vi "지진계측기(교수님 코드)_AI 및 DI 추가 스위치 제어.vi"() -> ()   [LabVIEW 2021]
uses:
  <vilib>/DAQmx/read.llb/DAQmx Read (Digital U8 1Chan 1Samp).vi
  <vilib>/DAQmx/read.llb/DAQmx Read (Analog 1D DBL 1Chan NSamp).vi
  <vilib>/Analysis/baseanly.llb/Mean (DBL).vi
  <vilib>/DAQmx/create/channels.llb/DAQmx Create Channel (AI-Voltage-Basic).vi
  <vilib>/DAQmx/configure/timing.llb/DAQmx Timing (Sample Clock).vi
  <vilib>/DAQmx/create/channels.llb/DAQmx Create Channel (DI-Digital Input).vi
  <vilib>/DAQmx/miscellaneous.llb/DAQmx Fill In Error Info.vi
  <vilib>/Analysis/NI_AALBase.lvlib
panel:
  out "문자열":string
  out "알람발생":bool
  in  "시작":bool
  out "웨이브폼 차트":dbl(graph)
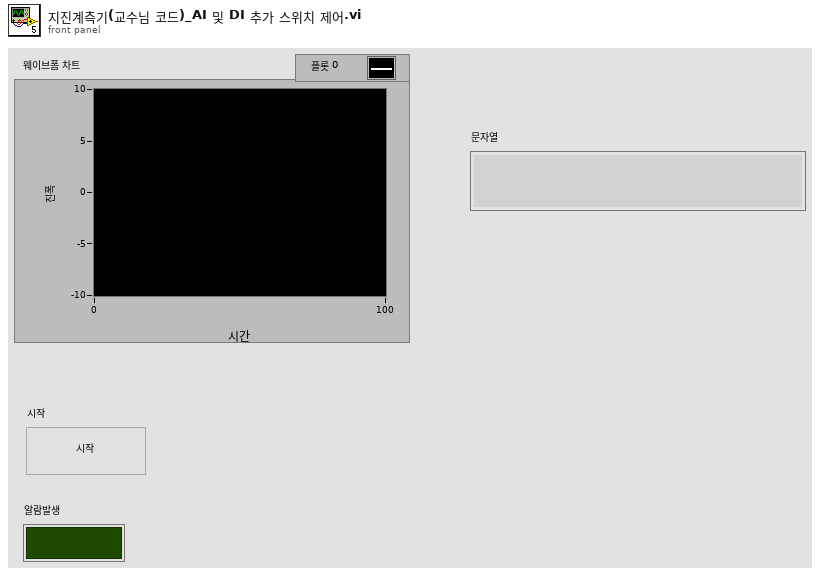
[diagram p1: front panel]
types:
  T1 = enum16{"초기화", "대기", "감지 시작", "알람 발생", "알람 리셋", "정지"}
  T2 = cluster{"AI":refnum<k21>, "DI":refnum<k21>, "알람 발생":bool, "데이터":dbl, "알람 데이터":string}
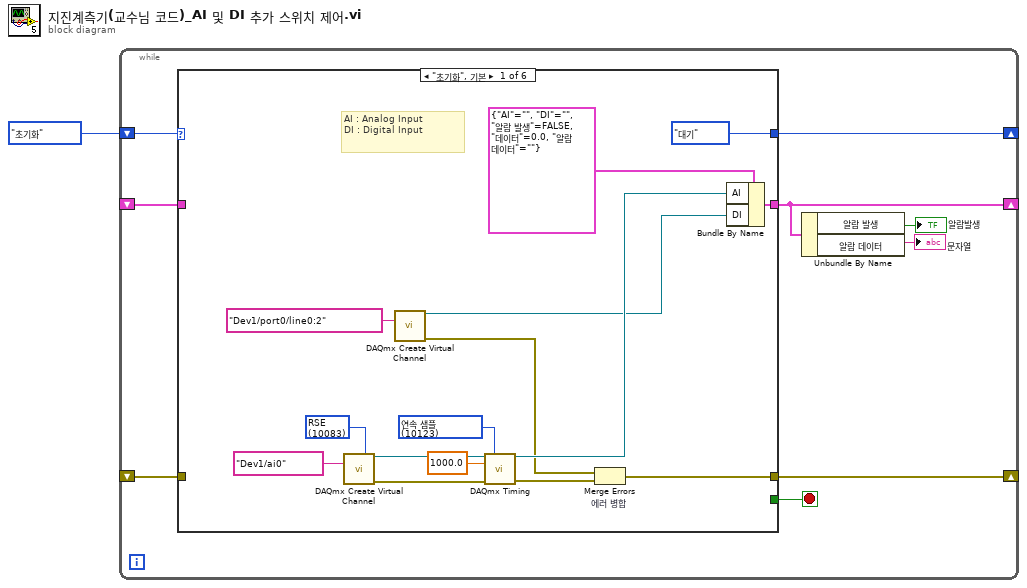
[diagram p0: block diagram]
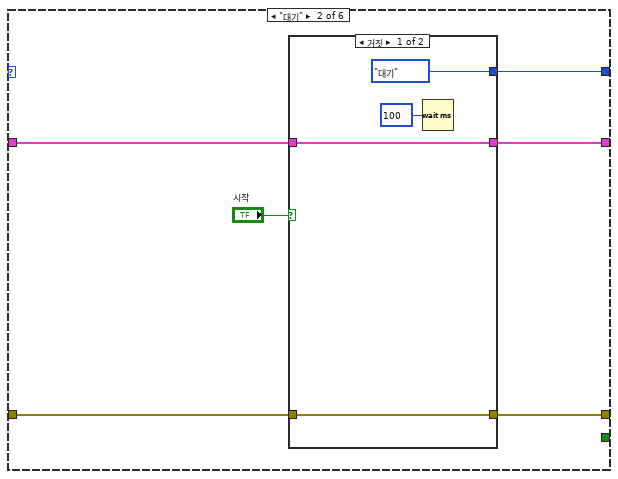
[diagram p2: hidden frame]
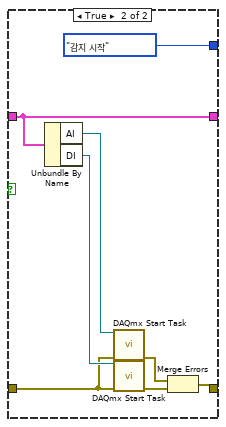
[diagram p3: hidden frame]
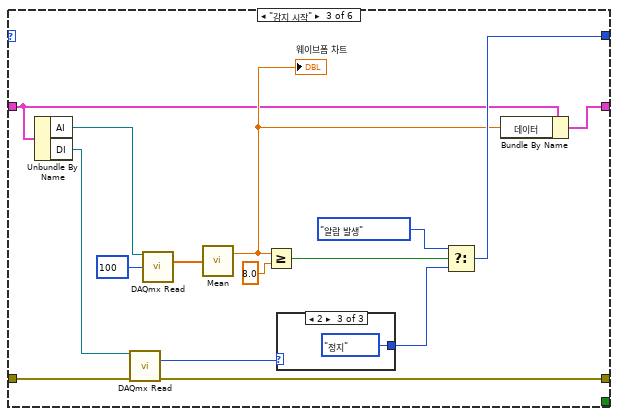
[diagram p4: hidden frame]
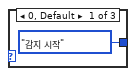
[diagram p5: hidden frame]
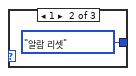
[diagram p6: hidden frame]
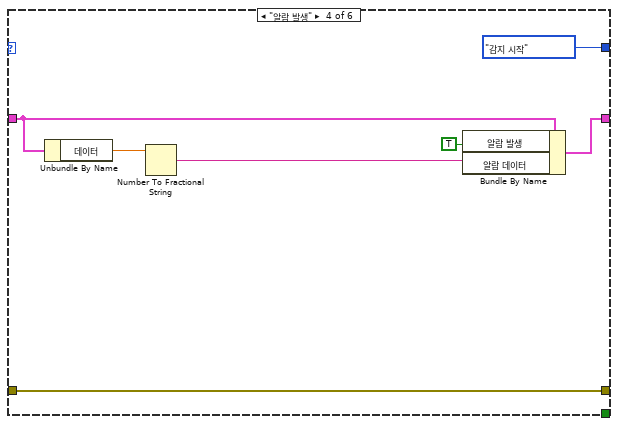
[diagram p7: hidden frame]
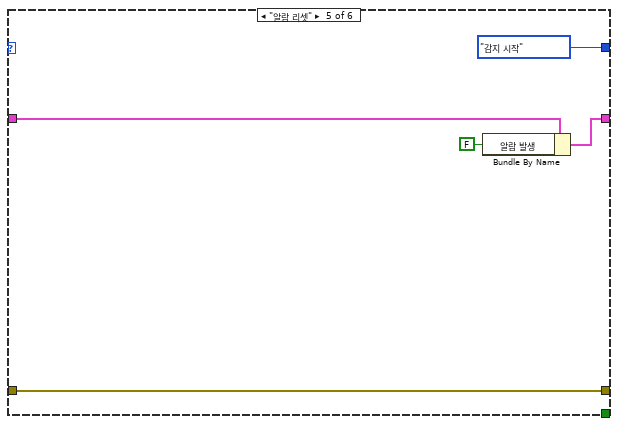
[diagram p8: hidden frame]
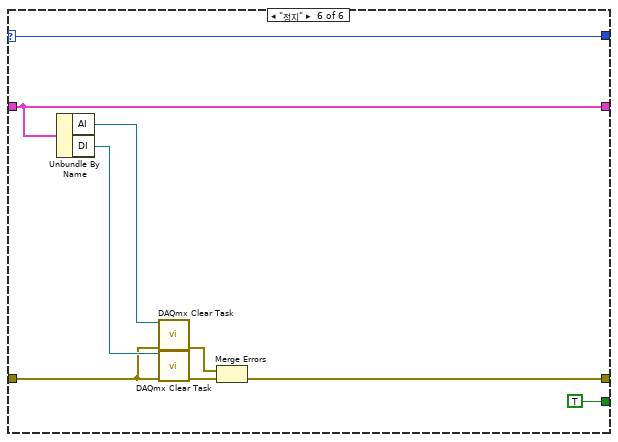
[diagram p9: hidden frame]
diagram:
  n1 = while {
    shift-right: [w3] -> _
    shift-left: T1."초기화" -> [w10]
    shift-right: [w7] -> _
    shift-left: _ -> [w9]
    shift-right: [w2] -> _
    shift-left: _ -> [w8]
    stop <- w5 stop-if-true
    n2 = case shown="\"초기화\", 기본" w10 {
      selector: w10 -> [_ _ _ _ _ w82]
      tunnel: [T1."대기" w29 w58 T1."감지 시작" T1."감지 시작" w82] -> w3
      tunnel: [w18 w27 w53 w67 w71 w80] -> w7
      tunnel: w9 -> [_ w30 w50 w64 w72 w80]
      tunnel: w8 -> [_ w28 w45 w65 w69 w77]
      tunnel: [w15 w26 w44 w65 w69 w74] -> w2
      tunnel: [_ _ _ _ _ TRUE] -> w5
      frame "초기화", Default {
        w21 = 10123 items=["유한 샘플"=10178, "연속 샘플"=10123, "하드웨어 타이밍에 의한 단일 포인트"=12522] ("sample mode")
        w22 = 10083 items=["기본"=-1, "RSE"=10083, "NRSE"=10078, "차동"=10106, "유사 차동"=12529] ("input terminal configuration")
        # "AI : Analog Input\nDI : Digital Input"
        n3 = call-poly <vilib>:"DAQmx Create Virtual Channel.vi"("input terminal configuration"=w22, "physical channels"=tag "Dev1/ai0") -> ("task out"=w25:refnum<k21>, "error out"=w24:errorcluster)  [unwired: 12 in]
        n4 = call-poly <vilib>:"DAQmx Create Virtual Channel.vi"("lines"=tag "Dev1/port0/line0:2") -> ("task out"=w13:refnum<k21>, "error out"=w11:errorcluster)  [unwired: 13 in]
        n5 = call-poly <vilib>:"DAQmx Timing.vi"("task/channels in"=w25, "sample mode"=w21, "rate"=1000.0, "error in"=w24) -> ("task out"=w17:refnum<k21>, "error out"=w12:errorcluster)  [unwired: 10 in]
        n6 = Merge Errors "에러 병합"(w11, w12) -> (w15:errorcluster)
        n7 = Bundle By Name(cluster=T2 {"AI"="", "DI"="", "알람 발생"=FALSE, "데이터"=0.0, "알람 데이터"=""}, "AI"=w17, "DI"=w13) -> (w18:T2)
      }
      frame "대기" {
        n8 = case shown="거짓" "시작" {
          tunnel: w30 -> [w35 w42]
          tunnel: [T1."대기" T1."감지 시작"] -> w29
          tunnel: w28 -> [w34 w36]
          tunnel: [w35 w42] -> w27
          tunnel: [w34 w37] -> w26
          frame False {
            n9 = Wait (ms)(milliseconds to wait=u32 100 ("대기 시간 (ms)")) -> ()  [unwired: 1 out]
          }
          frame True {
            n10 = Unbundle By Name(w42) -> ("AI"=w43:refnum<k21>, "DI"=w40:refnum<k21>)
            n11 = call <vilib>:"DAQmx Start Task.vi"("task/channels in"=w43, "error in"=w36) -> ("error out"=w38:errorcluster)  [unwired: 12 in, 1 out]
            n12 = call <vilib>:"DAQmx Start Task.vi"("task/channels in"=w40, "error in"=w36) -> ("error out"=w39:errorcluster)  [unwired: 12 in, 1 out]
            n13 = Merge Errors(w38, w39) -> (w37:errorcluster)
          }
        }
      }
      frame "감지 시작" {
        n14 = Unbundle By Name(w50) -> ("AI"=w51:refnum<k21>, "DI"=w49:refnum<k21>)
        n15 = call-poly <vilib>:"DAQmx Read.vi"("task/channels in"=w49, "error in"=w45) -> ("data"=w47:u8, "error out"=w44:errorcluster)  [unwired: 11 in, 1 out]
        n16 = call-poly <vilib>:"DAQmx Read.vi"("task/channels in"=w51, "number of samples per channel"=100) -> ("data"=w56:dbl[])  [unwired: 11 in, 2 out]
        n17 = call-poly <vilib>:"Mean.vi"("X"=w56) -> ("mean"=w52:dbl)  [unwired: 1 out]
        "웨이브폼 차트" <- w52
        n18 = Greater Or Equal?(x=w52, y=8.0) -> (x >= y?=w48:bool)
        n19 = case shown="2" w47 {
          tunnel: [T1."감지 시작" T1."알람 리셋" T1."정지"] -> w46
          frame 0, Default {
          }
          frame 1 {
          }
          frame 2 {
          }
        }
        n20 = Select(t=T1."알람 발생", s=w48, f=w46) -> (s? t:f=w58:T1)
        n21 = Bundle By Name(cluster=w50, "데이터"=w52) -> (w53:T2)
      }
      frame "알람 발생" {
        n22 = Unbundle By Name(w64) -> ("데이터"=w63:dbl)
        n23 = Number To Fractional String(number=w63) -> (F-format string=w62:string)  [unwired: 3 in]
        n24 = Bundle By Name(cluster=w64, "알람 발생"=TRUE, "알람 데이터"=w62) -> (w67:T2)
      }
      frame "알람 리셋" {
        n25 = Bundle By Name(cluster=w72, "알람 발생"=FALSE) -> (w71:T2)
      }
      frame "정지" {
        n26 = Unbundle By Name(w80) -> ("AI"=w79:refnum<k21>, "DI"=w78:refnum<k21>)
        n27 = call <vilib>:"DAQmx Clear Task.vi"("task in"=w79, "error in"=w77) -> ("error out"=w75:errorcluster)  [unwired: 13 in]
        n28 = call <vilib>:"DAQmx Clear Task.vi"("task in"=w78, "error in"=w77) -> ("error out"=w76:errorcluster)  [unwired: 13 in]
        n29 = Merge Errors(w75, w76) -> (w74:errorcluster)
      }
    }
    n30 = Unbundle By Name(w7) -> ("알람 발생"=→"알람발생":bool, "알람 데이터"=→"문자열":string)
  }
